vi "Perform Action.vi"(8 "error in (no error)":errorcluster, 10 "Input":variant, 11 "Read All CFG in":refnum<class "Read All CFG.lvclass">) -> (0 "error out":errorcluster, 2 "Output":variant, 3 "Read All CFG out":refnum<class "Read All CFG.lvclass">)   [LabVIEW 2023, in "NEO480HTA.lvlib" / "Read All CFG.lvclass"]
uses:
  Read All CFG.lvclass
  XNET/XNET Base CFG/XNET Base CFG.lvclass/XNET Base CFG.ctl
  <vilib>/xnet/xnet.llb/XNET Read (Frame CAN).vi
  <vilib>/ErrorRing/Error Ring.xnode
  XNET/XNET Base CFG/XNET Base CFG.lvclass
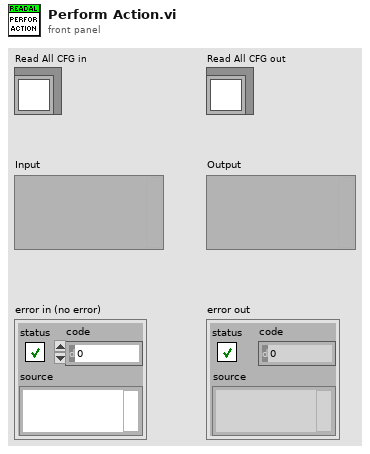
[diagram p1: front panel]
types:
  T1 = enum16{"Default", "Dew Point", "Pressure", "Temperature", "Sensor Status", "Dew Point Raw", "Absolute Humidity", "C H20"}
  T2 = typedef "XNET Frame CAN.ctl" = cluster{"timestamp":timestamp, "payload":u8[], "identifier":u32, "type":T3, "extended?":bool, "echo?":bool}
  T3 = typedef "XNET Frame Type CAN.ctl" = u8
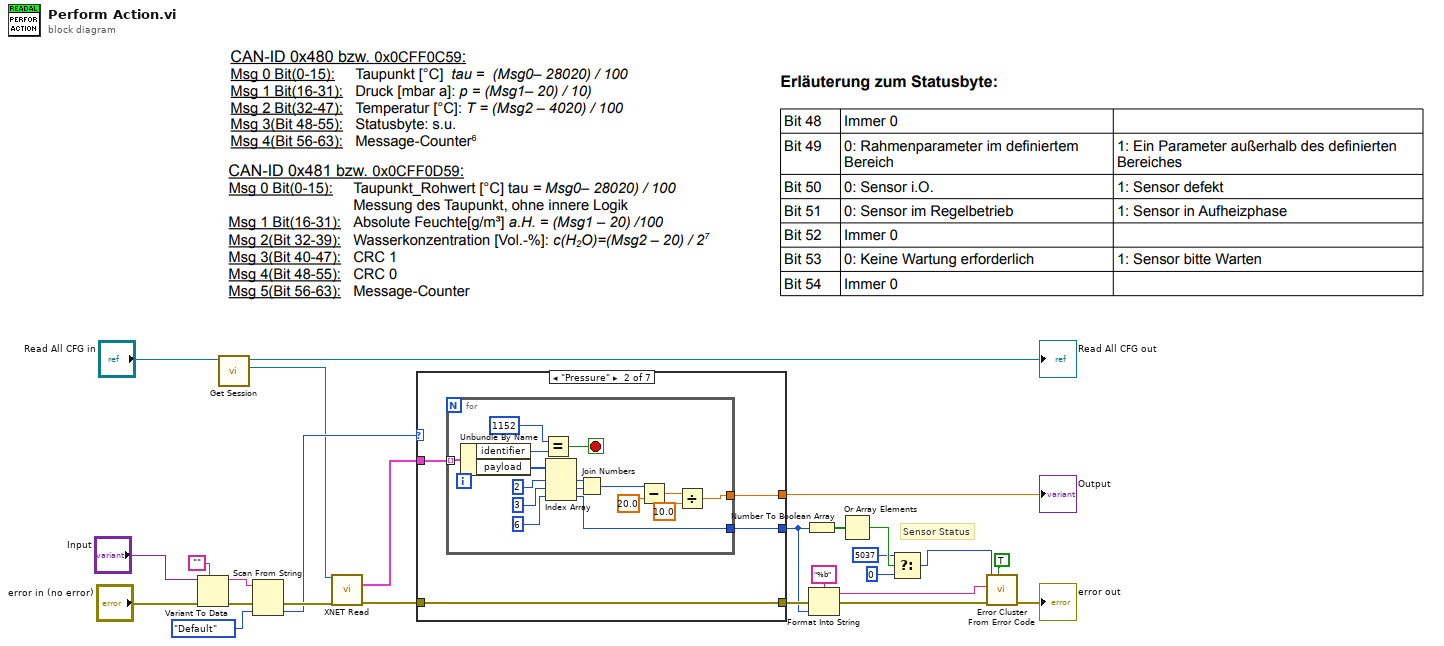
[diagram p0: block diagram]
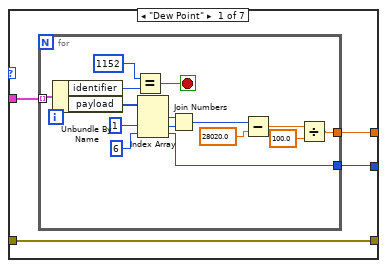
[diagram p2: hidden frame]
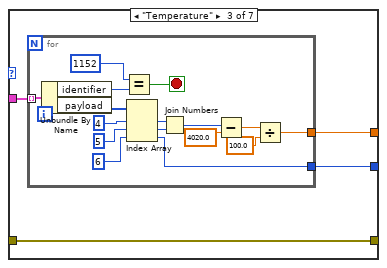
[diagram p3: hidden frame]
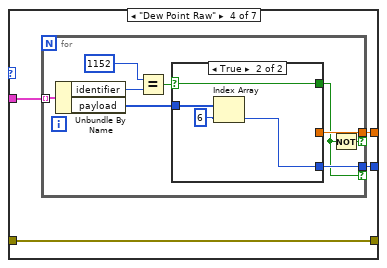
[diagram p4: hidden frame]
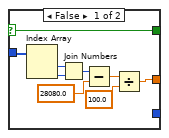
[diagram p5: hidden frame]
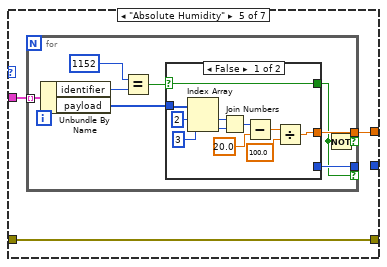
[diagram p6: hidden frame]
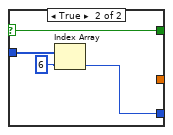
[diagram p7: hidden frame]
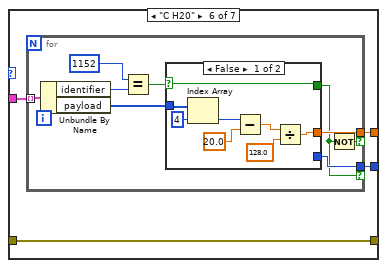
[diagram p8: hidden frame]
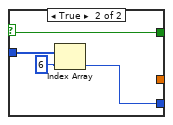
[diagram p9: hidden frame]
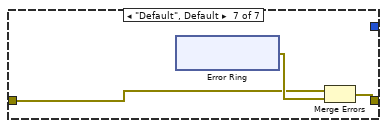
[diagram p10: hidden frame]
diagram:
  # "Sensor Status"
  n1 = Variant To Data(error in="error in (no error)", type="" ("Empty String Constant"), Variant="Input") -> (data=w19:string, error out=w25:errorcluster)
  n2 = call "Get Session.vi"("XNET Base CFG in"="Read All CFG in") -> ("Session"=w1:refnum<k21>, "XNET Base CFG out"=→"Read All CFG out":refnum<class "Read All CFG.lvclass">)  [unwired: 8 in, 1 out]
  n3 = Scan From String(input string=w19, error in=w25, default 1=T1."Default") -> (error out=w21:errorcluster, output 1=w4:T1)  [unwired: 2 in, 2 out]
  n4 = call-poly <vilib>:"XNET Read.vi"("session in"=w1, "error in (no error)"=w21) -> ("data"=w18:T2[], "error out"=w22:errorcluster)  [unwired: 12 out]
  n5 = case shown="\"Pressure\"" w4 {
    tunnel: w22 -> [w27 w47 w66 w87 w112 w139 w165]
    tunnel: [w27 w47 w66 w87 w112 w139 w164] -> w7
    tunnel: w18 -> [w30 w49 w69 w89 w114 w142 _]
    tunnel: [w29 w48 w68 w86 w113 w140 _] -> w17
    tunnel: [w28 w46 w67 w88 _ w141 _] -> w5
    frame "Dew Point" {
      n6 = for {
        tunnel: w30 -> [w45] mode=indexing
        tunnel: [w36] -> w29
        tunnel: [w32] -> w28
        stop <- w35 stop-if-true
        n7 = Unbundle By Name(w45) -> ("identifier"=w44:u32, "payload"=w40:u8[])
        n8 = Equal?(x=u32 1152, y=w44) -> (x = y?=w35:bool)
        n9 = Index Array(array=w40, index #2=1 ("index"), index #3=6 ("index")) -> (element #1=w39:u8, element #2=w38:u8, element #3=w32:u8)  [unwired: 1 in]
        n10 = Join Numbers(hi=w39, lo=w38) -> ((hi.lo)=w37:u16)
        n11 = Subtract(x=w37, y=28020.0) -> (x-y=w41:dbl)
        n12 = Divide(x=w41, y=100.0) -> (x/y=w36:dbl)
      }
    }
    frame "Pressure" {
      n13 = for {
        tunnel: w49 -> [w65] mode=indexing
        tunnel: [w54] -> w48
        tunnel: [w50] -> w46
        stop <- w61 stop-if-true
        n14 = Unbundle By Name(w65) -> ("identifier"=w64:u32, "payload"=w62:u8[])
        n15 = Equal?(x=u32 1152, y=w64) -> (x = y?=w61:bool)
        n16 = Index Array(array=w62, index #1=2 ("index"), index #2=3 ("index"), index #3=6 ("index")) -> (element #1=w57:u8, element #2=w56:u8, element #3=w50:u8)
        n17 = Join Numbers(hi=w57, lo=w56) -> ((hi.lo)=w55:u16)
        n18 = Subtract(x=w55, y=20.0) -> (x-y=w58:dbl)
        n19 = Divide(x=w58, y=10.0) -> (x/y=w54:dbl)
      }
    }
    frame "Temperature" {
      n20 = for {
        tunnel: w69 -> [w85] mode=indexing
        tunnel: [w75] -> w68
        tunnel: [w71] -> w67
        stop <- w81 stop-if-true
        n21 = Unbundle By Name(w85) -> ("identifier"=w84:u32, "payload"=w82:u8[])
        n22 = Equal?(x=u32 1152, y=w84) -> (x = y?=w81:bool)
        n23 = Index Array(array=w82, index #1=4 ("index"), index #2=5 ("index"), index #3=6 ("index")) -> (element #1=w78:u8, element #2=w77:u8, element #3=w71:u8)
        n24 = Join Numbers(hi=w78, lo=w77) -> ((hi.lo)=w76:u16)
        n25 = Subtract(x=w76, y=4020.0) -> (x-y=w79:dbl)
        n26 = Divide(x=w79, y=100.0) -> (x/y=w75:dbl)
      }
    }
    frame "Dew Point Raw" {
      n27 = for {
        tunnel: w89 -> [w98] mode=indexing
        tunnel: [w93] -> w88 if=w91
        tunnel: [w92] -> w86 if=w90
        n28 = Unbundle By Name(w98) -> ("identifier"=w97:u32, "payload"=w95:u8[])
        n29 = Equal?(x=u32 1152, y=w97) -> (x = y?=w94:bool)
        n30 = case shown="True" w94 {
          selector: w94 -> [w99 w108]
          tunnel: w95 -> [w107 w111]
          tunnel: [_ w109] -> w93
          tunnel: [w100 _] -> w92
          tunnel: [w99 w108] -> w91
          frame False {
            n31 = Index Array(array=w107) -> (element #1=w106:u8, element #2=w105:u8)  [unwired: 2 in]
            n32 = Join Numbers(hi=w106, lo=w105) -> ((hi.lo)=w104:u16)
            n33 = Subtract(x=w104, y=28080.0) -> (x-y=w102:dbl)
            n34 = Divide(x=w102, y=100.0) -> (x/y=w100:dbl)
          }
          frame True {
            n35 = Index Array(array=w111, index=6) -> (element=w109:u8)
          }
        }
        n36 = Not(x=w91) -> (.not. x?=w90:bool)
      }
    }
    frame "Absolute Humidity" {
      n37 = for {
        tunnel: w114 -> [w123] mode=indexing
        tunnel: [w118] -> _ if=w115
        tunnel: [w117] -> w113 if=w116
        n38 = Unbundle By Name(w123) -> ("identifier"=w122:u32, "payload"=w120:u8[])
        n39 = Equal?(x=u32 1152, y=w122) -> (x = y?=w119:bool)
        n40 = case shown="False" w119 {
          selector: w119 -> [w124 w135]
          tunnel: w120 -> [w134 w138]
          tunnel: [_ w136] -> w118
          tunnel: [w127 _] -> w117
          tunnel: [w124 w135] -> w115
          frame False {
            n41 = Index Array(array=w134, index #1=2 ("index"), index #2=3 ("index")) -> (element #1=w133:u8, element #2=w132:u8)
            n42 = Join Numbers(hi=w133, lo=w132) -> ((hi.lo)=w131:u16)
            n43 = Subtract(x=w131, y=20.0) -> (x-y=w129:dbl)
            n44 = Divide(x=w129, y=100.0) -> (x/y=w127:dbl)
          }
          frame True {
            n45 = Index Array(array=w138, index=6) -> (element=w136:u8)
          }
        }
        n46 = Not(x=w115) -> (.not. x?=w116:bool)
      }
    }
    frame "C H20" {
      n47 = for {
        tunnel: w142 -> [w151] mode=indexing
        tunnel: [w147] -> w141 if=w144
        tunnel: [w146] -> w140 if=w143
        n48 = Unbundle By Name(w151) -> ("identifier"=w150:u32, "payload"=w148:u8[])
        n49 = Equal?(x=u32 1152, y=w150) -> (x = y?=w145:bool)
        n50 = case shown="False" w145 {
          selector: w145 -> [w152 w160]
          tunnel: w148 -> [w159 w163]
          tunnel: [_ w161] -> w147
          tunnel: [w155 _] -> w146
          tunnel: [w152 w160] -> w144
          frame False {
            n51 = Index Array(array=w159, index=4) -> (element=w153:u8)
            n52 = Subtract(x=w153, y=20.0) -> (x-y=w157:dbl)
            n53 = Divide(x=w157, y=128.0) -> (x/y=w155:dbl)
          }
          frame True {
            n54 = Index Array(array=w163, index=6) -> (element=w161:u8)
          }
        }
        n55 = Not(x=w144) -> (.not. x?=w143:bool)
      }
    }
    frame "Default", Default {
      n56 = xnode "Error Ring"() -> ("error out"=w166:errorcluster)
      n57 = Merge Errors(w165, w166) -> (w164:errorcluster)
    }
  }
  "Output" <- w17
  n58 = Number To Boolean Array(number=w5) -> (Boolean array=w13:bool[])
  n59 = Format Into String(format string="%b", error in=w7, w5) -> (resulting string=w14:string, error out=w15:errorcluster)  [unwired: 1 in]
  n60 = Or Array Elements(Boolean array=w13) -> (logical OR=w12:bool)
  n61 = Select(t=5037, s=w12, f=0) -> (s? t:f=w16:i32)
  n62 = call <vilib>:"Error Cluster From Error Code.vi"("show call chain? (False)"=TRUE, "error in (no error)"=w15, "error message (\"\")"=w14, "error code (0)"=w16) -> ("error out"=→"error out":errorcluster)  [unwired: 5 in]
